vi "ArthOps.vi"() -> ()   [LabVIEW 2026]
panel:
  out "x-5":dbl
  out "floor(x): largest int <= x":dbl
  out "x+1":dbl
  out "x*2^n":dbl
  in  "x":dbl
  in  "y":dbl
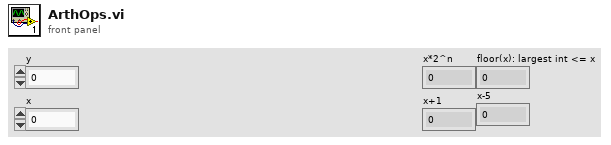
[diagram p1: front panel]
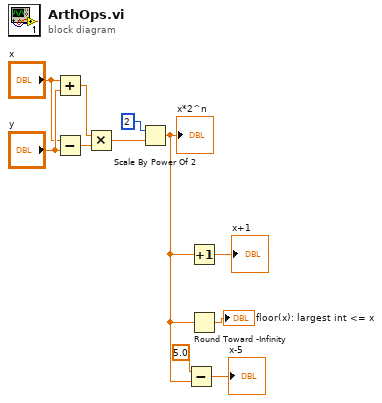
[diagram p0: block diagram]
diagram:
  n1 = Add(x="x", y="y") -> (x+y=w9:dbl)
  n2 = Subtract(x="x", y="y") -> (x-y=w8:dbl)
  n3 = Multiply(x=w9, y=w8) -> (x*y=w7:dbl)
  n4 = Scale By Power Of 2(n=i16 2, x=w7) -> (x*2^n=w2:dbl)
  "x*2^n" <- w2
  n5 = Subtract(x=5.0, y=w2) -> (x-y=→"x-5":dbl)
  n6 = Increment(x=w2) -> (x+1=→"x+1":dbl)
  n7 = Round Toward -Infinity(1:w2) -> (0:→"floor(x): largest int <= x":dbl)
